vi "Finish.vi"   [LabVIEW 2017]
doc: "This VI is called during exit. It can be used to close I/O refnums, save collected data, etc."
uses:
  <vilib>/Rock Robotics/WPI/Utilities/WPI_GetSetVariantRefNum.vi
types:
  T1 = typedef "WPI_CompressorDevRef.ctl" = cluster{"DevStatus":errorcluster, "Pneumatics Control Module":u8}
  T2 = typedef "WPI_MotorControlDeviceRef.ctl" = cluster{"DeviceStatus":errorcluster, "Type":T3, "PWM":cluster{"PWM Channel":T4, "DeadBand":T5}, "CAN":cluster{"Device Number":u8, "SetOutput VI Ref":variant, "GetOutput VI Ref":variant, "Enable VI Ref":variant, "Disable VI Ref":variant, "Data":variant}, "Invert":bool, "DIO PWM":cluster{"PWM \"Enable\" Channel":T4, "DIOChannel":T6, "PWM Rate":dbl}}
  T3 = typedef "WPI_MotorControlType.ctl" = enum16{"PWM", "CAN", "DIO PWM"}
  T4 = typedef "FPGA_DIOPWMChannel.ctl" = enum8{"PWM 0", "PWM 1", "PWM 2", "PWM 3", "PWM 4", "PWM 5", "PWM 6", "PWM 7", "PWM 8", "PWM 9", "PWM MXP 0", "PWM MXP 1", "PWM MXP 2", "PWM MXP 3", "PWM MXP 4", "PWM MXP 5", "PWM MXP 6", "PWM MXP 7", "PWM MXP 8", "PWM MXP 9", "Invalid"}
  T5 = typedef "WPI_PWMDeadband.ctl" = cluster{"Name":string, "maxPositivePwm":i32, "minPositivePwm":i32, "centerPwm":i32, "maxNegativePwm":i32, "minNegativePwm":i32, "angularRange":u16}
  T6 = typedef "FPGA_DIOChannel.ctl" = enum8{"DIO 0", "DIO 1", "DIO 2", "DIO 3", "DIO 4", "DIO 5", "DIO 6", "DIO 7", "DIO 8", "DIO 9", "DIO MXP 0", "DIO MXP 1", "DIO MXP 2", "DIO MXP 3", "DIO MXP 4", "DIO MXP 5", "DIO MXP 6", "DIO MXP 7", "DIO MXP 8", "DIO MXP 9", "DIO MXP 10", "DIO MXP 11", "DIO MXP 12", "DIO MXP 13", "DIO MXP 14", "DIO MXP 15", "SPI Port CS1", "SPI Port CS2", "SPI Port CS3", "SPI Port MISO", "SPI Port MOSI", "Invalid"}
  T7 = typedef "WPI_EncoderDevRef.ctl" = cluster{"DevStatus":errorcluster, "EncoderIndex":T8, "CounterIndex":T9, "DistancePerCount":dbl, "Decoding Type":T10}
  T8 = typedef "FPGA_EncoderIdx.ctl" = enum8{"Enc 0", "Enc 1", "Enc 2", "Enc 3", "Enc 4", "Enc 5", "Enc 6", "Enc 7", "Invalid"}
  T9 = typedef "FPGA_CounterCtrSystemIndex.ctl" = enum8{"Ctr 0", "Ctr 1", "Ctr 2", "Ctr 3", "Ctr 4", "Ctr 5", "Ctr 6", "Ctr 7", "Invalid"}
  T10 = typedef "WPI_EncoderType.ctl" = enum16{"1x", "2x", "4x"}
  T11 = typedef "WPI_RelayDevRef.ctl" = cluster{"DevStatus":errorcluster, "Relay Channel":T12, "Relay Direction":T13}
  T12 = typedef "FPGA_DIORelayChannel.ctl" = enum8{"Relay 0", "Relay 1", "Relay 2", "Relay 3", "Invalid"}
  T13 = typedef "WPI_RelayDirection.ctl" = enum16{"Both directions", "Forward only", "Reverse only"}
  T14 = typedef "WPI_DigitalInputDevRef.ctl" = cluster{"DevStatus":errorcluster, "DIO Channel":T6}
  T15 = typedef "WPI_RobotDriveDevRef.ctl" = cluster{"DevStatus":errorcluster, "Motors[]":T2[], "Square Inputs":bool, "Max Output":dbl}
  T16 = typedef "WPI_JoystickDevRef.ctl" = cluster{"Device":T17}
  T17 = typedef "WPI_JoystickDeviceEnum.ctl" = enum16{"USB 0", "USB 1", "USB 2", "USB 3", "USB 4", "USB 5"}
  T18 = typedef "WPI_SolenoidDevRef.ctl" = cluster{"DevStatus":errorcluster, "Pneumatics Control Module":u8, "Forward Solenoid Channel":T19, "Reverse Solenoid Channel":T19}
  T19 = typedef "WPI_SolenoidChannel.ctl" = enum8{"Solenoid 0", "Solenoid 1", "Solenoid 2", "Solenoid 3", "Solenoid 4", "Solenoid 5", "Solenoid 6", "Solenoid 7", "Invalid"}
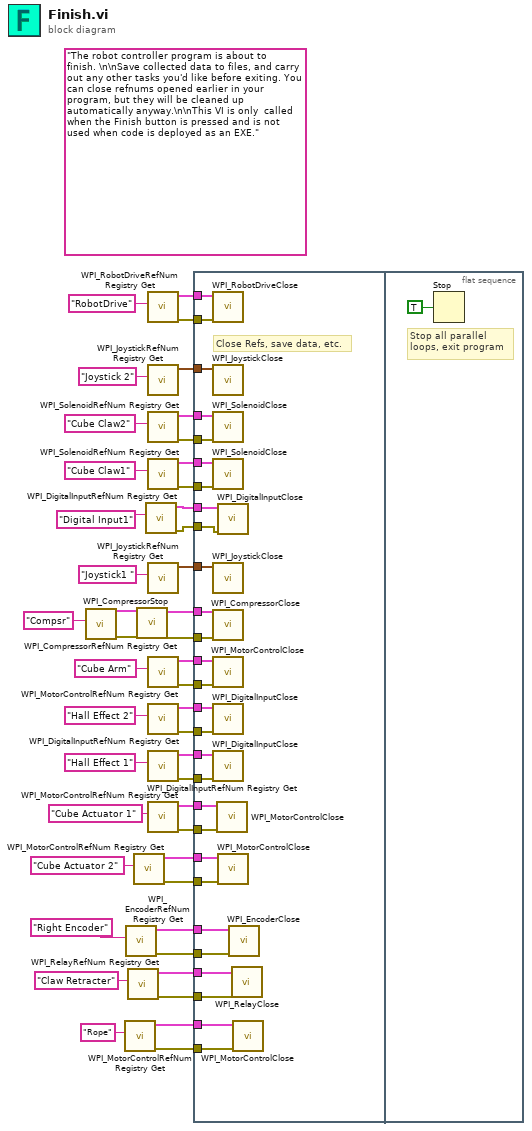
[diagram p0: block diagram]
diagram:
  (unwired) "The robot controller program is about to finish. \n\nSave collected data to files, and carry out any other tasks you'd like before exiting. You can close refnums opened earlier in your program, but they will be cleaned up automatically anyway.\n\nThis VI is only  called when the Finish button is pressed and is not used when code is deployed as an EXE."
  n1 = call <vilib>:"WPI_CompressorRefNum Registry Get.vi"("refnum name"="Compsr") -> ("error out"=w6:errorcluster, "CompressorDevRef"=w7:T1)  [unwired: 9 in]
  n2 = call <vilib>:"WPI_MotorControlRefNum Registry Get.vi"("refnum name"="Rope") -> ("error out"=w2:errorcluster, "MotorControlDevRef"=w3:T2)  [unwired: 9 in]
  n3 = call <vilib>:"WPI_EncoderRefNum Registry Get.vi"("refnum name"="Right Encoder") -> ("error out"=w14:errorcluster, "EncoderDevRef"=w16:T7)  [unwired: 9 in]
  n4 = call <vilib>:"WPI_RelayRefNum Registry Get.vi"("refnum name"="Claw Retracter") -> ("error out"=w12:errorcluster, "RelayDevRef"=w13:T11)  [unwired: 9 in]
  n5 = call <vilib>:"WPI_MotorControlRefNum Registry Get.vi"("refnum name"="Cube Actuator 2") -> ("error out"=w19:errorcluster, "MotorControlDevRef"=w20:T2)  [unwired: 9 in]
  n6 = call <vilib>:"WPI_CompressorStop.vi"("error in (no error)"=w6, "CompressorDevRef"=w7) -> ("error out"=w4:errorcluster, "CompressorDevRef"=w5:T1)  [unwired: 8 in]
  n7 = call <vilib>:"WPI_DigitalInputRefNum Registry Get.vi"("refnum name"="Digital Input1") -> ("error out"=w8:errorcluster, "DigitalInputDevRef"=w9:T14)  [unwired: 9 in]
  n8 = call <vilib>:"WPI_RobotDriveRefNum Registry Get.vi"("refnum name"="RobotDrive") -> ("error out"=w40:errorcluster, "RobotDriveDevRef"=w41:T15)  [unwired: 9 in]
  n9 = call <vilib>:"WPI_JoystickRefNum Registry Get.vi"("refnum name"="Joystick 2") -> ("JoystickDevRef"=w44:T16)  [unwired: 1 in, 9 out]
  n10 = call <vilib>:"WPI_SolenoidRefNum Registry Get.vi"("refnum name"="Cube Claw2") -> ("error out"=w25:errorcluster, "SolenoidDevRef"=w26:T18)  [unwired: 9 in]
  n11 = call <vilib>:"WPI_SolenoidRefNum Registry Get.vi"("refnum name"="Cube Claw1") -> ("error out"=w27:errorcluster, "SolenoidDevRef"=w28:T18)  [unwired: 9 in]
  n12 = call <vilib>:"WPI_JoystickRefNum Registry Get.vi"("refnum name"="Joystick1 ") -> ("JoystickDevRef"=w43:T16)  [unwired: 1 in, 9 out]
  n13 = call <vilib>:"WPI_MotorControlRefNum Registry Get.vi"("refnum name"="Cube Arm") -> ("error out"=w31:errorcluster, "MotorControlDevRef"=w32:T2)  [unwired: 9 in]
  n14 = call <vilib>:"WPI_DigitalInputRefNum Registry Get.vi"("refnum name"="Hall Effect 2") -> ("error out"=w34:errorcluster, "DigitalInputDevRef"=w35:T14)  [unwired: 9 in]
  n15 = call <vilib>:"WPI_DigitalInputRefNum Registry Get.vi"("refnum name"="Hall Effect 1") -> ("error out"=w37:errorcluster, "DigitalInputDevRef"=w38:T14)  [unwired: 9 in]
  n16 = call <vilib>:"WPI_MotorControlRefNum Registry Get.vi"("refnum name"="Cube Actuator 1") -> ("error out"=w21:errorcluster, "MotorControlDevRef"=w22:T2)  [unwired: 9 in]
  n17 = flat-sequence {
    tunnel: w44 -> [w73]
    tunnel: w43 -> [w72]
    tunnel: w41 -> [w71]
    tunnel: w40 -> [w70]
    tunnel: w38 -> [w69]
    tunnel: w37 -> [w68]
    tunnel: w35 -> [w67]
    tunnel: w34 -> [w66]
    tunnel: w32 -> [w65]
    tunnel: w31 -> [w64]
    tunnel: w28 -> [w63]
    tunnel: w27 -> [w62]
    tunnel: w26 -> [w61]
    tunnel: w25 -> [w60]
    tunnel: w22 -> [w59]
    tunnel: w21 -> [w58]
    tunnel: w20 -> [w57]
    tunnel: w19 -> [w56]
    tunnel: w16 -> [w55]
    tunnel: w14 -> [w54]
    tunnel: w13 -> [w53]
    tunnel: w12 -> [w52]
    tunnel: w9 -> [w51]
    tunnel: w8 -> [w50]
    tunnel: w5 -> [w49]
    tunnel: w4 -> [w48]
    tunnel: w3 -> [w47]
    tunnel: w2 -> [w46]
    frame #0 {
      # "Close Refs, save data, etc."
      n18 = call <vilib>:"WPI_RobotDriveClose.vi"("error in (no error)"=w70, "RobotDriveDevRef"=w71) -> ()  [unwired: 9 in, 1 out]
      n19 = call <vilib>:"WPI_JoystickClose.vi"("JoystickDevRef"=w73) -> ()  [unwired: 11 out]
      n20 = call <vilib>:"WPI_SolenoidClose.vi"("error in (no error)"=w60, "SolenoidDevRef"=w61) -> ()  [unwired: 9 in, 1 out]
      n21 = call <vilib>:"WPI_SolenoidClose.vi"("error in (no error)"=w62, "SolenoidDevRef"=w63) -> ()  [unwired: 9 in, 1 out]
      n22 = call <vilib>:"WPI_JoystickClose.vi"("JoystickDevRef"=w72) -> ()  [unwired: 11 out]
      n23 = call <vilib>:"WPI_CompressorClose.vi"("error in (no error)"=w48, "CompressorDevRef"=w49) -> ()  [unwired: 9 in, 1 out]
      n24 = call <vilib>:"WPI_MotorControlClose.vi"("error in"=w64, "MotorControlDevRef"=w65) -> ()  [unwired: 9 in, 1 out]
      n25 = call <vilib>:"WPI_DigitalInputClose.vi"("error in (no error)"=w66, "DigitalInputDevRef"=w67) -> ()  [unwired: 9 in, 1 out]
      n26 = call <vilib>:"WPI_DigitalInputClose.vi"("error in (no error)"=w68, "DigitalInputDevRef"=w69) -> ()  [unwired: 9 in, 1 out]
      n27 = call <vilib>:"WPI_MotorControlClose.vi"("error in"=w58, "MotorControlDevRef"=w59) -> ()  [unwired: 9 in, 1 out]
      n28 = call <vilib>:"WPI_DigitalInputClose.vi"("error in (no error)"=w50, "DigitalInputDevRef"=w51) -> ()  [unwired: 9 in, 1 out]
      n29 = call <vilib>:"WPI_MotorControlClose.vi"("error in"=w56, "MotorControlDevRef"=w57) -> ()  [unwired: 9 in, 1 out]
      n30 = call <vilib>:"WPI_EncoderClose.vi"("error in (no error)"=w54, "EncoderDevRef"=w55) -> ()  [unwired: 9 in, 1 out]
      n31 = call <vilib>:"WPI_RelayClose.vi"("error in (no error)"=w52, "RelayDevRef"=w53) -> ()  [unwired: 9 in, 1 out]
      n32 = call <vilib>:"WPI_MotorControlClose.vi"("error in"=w46, "MotorControlDevRef"=w47) -> ()  [unwired: 9 in, 1 out]
    }
    frame #1 {
      # "Stop all parallel\nloops, exit program"
      n33 = Stop(stop? (T)=TRUE ("Quit")) -> ()
    }
  }
